vi "Interface2020.vi"() -> ()   [LabVIEW 2020]
panel:
  out "PREP PRESSURE":dynamicdata(graph)
  out "STM PRESSURE":dynamicdata(graph)
  out "udp recv raw":string
  # "Pressure Control Interface"
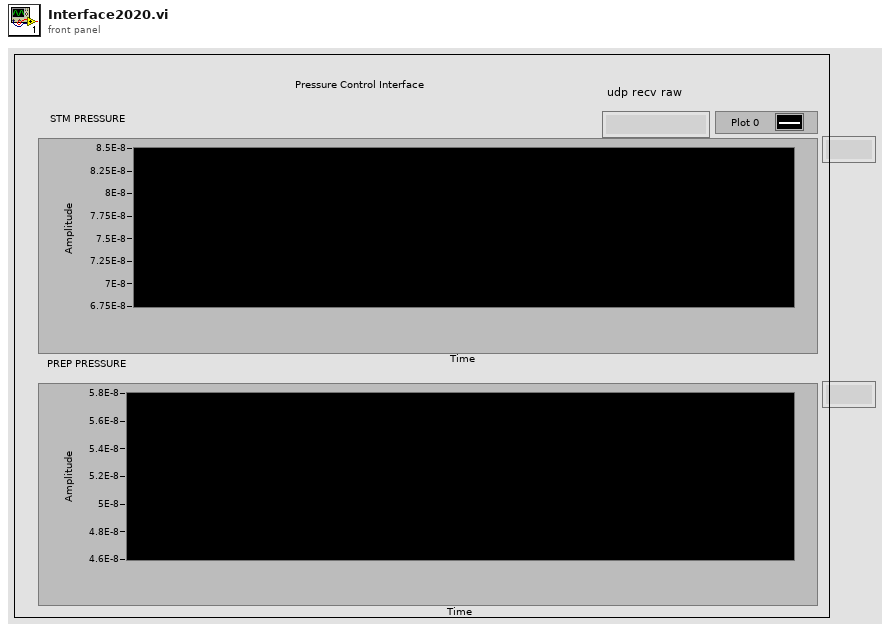
[diagram p1: front panel]
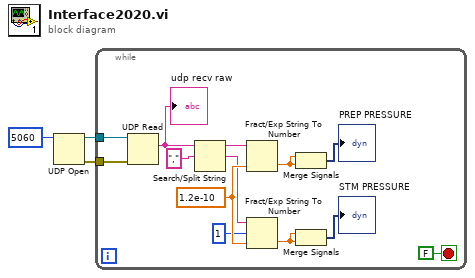
[diagram p0: block diagram]
diagram:
  n1 = UDP Open(11:u16 5060 ("port")) -> (port=w2:refnum<k16>, 0:w1:errorcluster)  [unwired: 4 in, 1 out]
  n2 = while {
    tunnel: w2 -> [w16]
    tunnel: w1 -> [w15]
    stop <- FALSE stop-if-true
    w9 = 1.2e-10
    n3 = UDP Read(connection ID=w16, 8:w15) -> (data out=w11:string)  [unwired: 2 in, 4 out]
    "udp recv raw" <- w11
    n4 = Search/Split String(string=w11, search string/char (-)=",") -> (substring before match=w7:string, match + rest of string=w4:string)  [unwired: 1 in, 1 out]
    n5 = Fract/Exp String To Number(string=w7, default (0 dbl)=w9) -> (number=w6:dbl)  [unwired: 2 in, 1 out]
    n6 = Fract/Exp String To Number(string=w4, offset=1, default (0 dbl)=w9) -> (number=w5:dbl)  [unwired: 1 in, 1 out]
    n7 = Merge Signals(w6, w6) -> (→"PREP PRESSURE":dynamicdata)
    n8 = Merge Signals(w5, w5) -> (→"STM PRESSURE":dynamicdata)
  }
